vi "Get Config Ref.vi"(8 "error in":errorcluster, 11 "Ex Nested in":refnum<class "SuperActor.lvclass">) -> (0 "error out":errorcluster, 2 "config ref":T1, 3 "Ex Nested out":refnum<class "SuperActor.lvclass">)   [LabVIEW 2015, in "SuperActor.lvclass"]
uses:
  SuperActor.lvclass
  <vilib>/Utility/config.llb/Config Data RefNum.ctl
  <vilib>/MSR Consulting, LLC/General Reuse/Session APIs/File Access/Config Data/Config Data.lvclass
  SuperActor.lvclass/SuperActor.ctl
  <vilib>/MSR Consulting, LLC/General Reuse/Session APIs/File Access/Config Data/Config Data.lvclass/Config Data.ctl
  <vilib>/Utility/config.llb/NI_LVConfig.lvlib
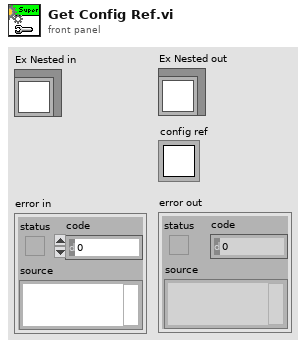
[diagram p1: front panel]
types:
  T1 = typedef "NI_LVConfig.lvlib/Config Data RefNum.ctl" = refnum<k1>
  T2 = typedef "Session - Root.lvclass/Session Handle.ctl" = refnum<data-value>
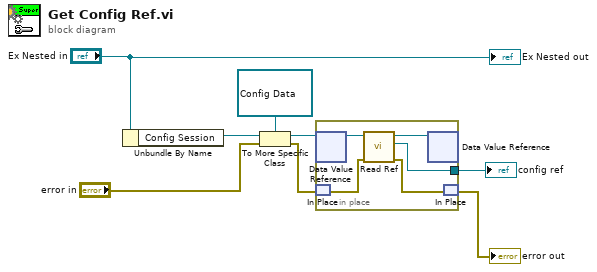
[diagram p0: block diagram]
diagram:
  n1 = Unbundle By Name("Ex Nested in") -> ("Config Session"=w7:T2)
  n2 = To More Specific Class(target class=refnum<data-value> refnum ("Config Session"), reference=w7, error in="error in") -> (specific class reference=w5:refnum<data-value>, error out=w4:errorcluster)
  n3 = in-place {
    in-place-border: [w10] -> w1
    n4 = in-place-dvr #1(w5) -> (w13:refnum<class "Config Data.lvclass">)  [unwired: 1 out]
    n5 = in-place-match #2(w4) -> (w11:errorcluster)
    n6 = call <vilib>:"Read Ref.vi"("error in"=w11, "Config Data in"=w13) -> ("error out"=w9:errorcluster, "config data"=w10:T1, "Config Data out"=w12:refnum<class "Config Data.lvclass">)  [unwired: 7 in]
    n7 = in-place-dvr #1(w12) -> ()  [unwired: 2 out]
    n8 = in-place-match #2(w9) -> (→"error out":errorcluster)
  }
  "config ref" <- w1
  "Ex Nested out" <- "Ex Nested in"
